vi "Set Message.vi"(8 "error in (no error)":errorcluster {"code" format="Error %.0f"}, 10 "Message":string, 11 "Progress Bar UI In":refnum<class "Progress Bar UI.lvclass">) -> (0 "error out":errorcluster {"code" format="Error %.0f"}, 3 "Progress Bar UI Out":refnum<class "Progress Bar UI.lvclass">)   [LabVIEW 2023, in "Progress Bar UI.lvclass"]
uses:
  Progress Bar UI.lvclass
  Progress Bar UI.lvclass/Progress Bar UI.ctl
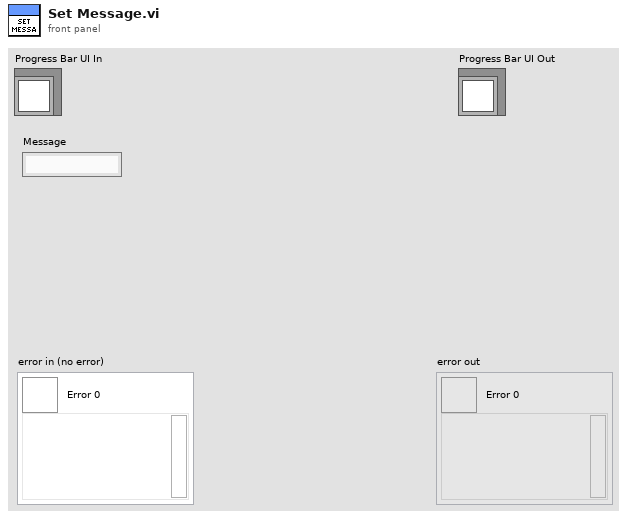
[diagram p1: front panel]
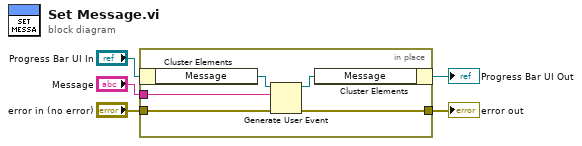
[diagram p0: block diagram]
diagram:
  n1 = in-place {
    in-place-border: "Message" -> [w8]
    in-place-border: "error in (no error)" -> [w7]
    in-place-border: [w6] -> w1
    n2 = in-place-cluster #1("Progress Bar UI In") -> ("Message"=w10:refnum<user-event>)
    n3 = Generate User Event(user event=w10, event data cluster=w8, error in=w7) -> (user event out=w9:refnum<user-event>, error out=w6:errorcluster)  [unwired: 1 in]
    n4 = in-place-cluster #1("Message"=w9) -> (→"Progress Bar UI Out":refnum<class "Progress Bar UI.lvclass">)
  }
  "error out" <- w1
